vi "varun weather simu.vi"() -> ()   [LabVIEW 2021]
panel:
  in  "stop":bool
  out "Temp Status":string
  out "Freeze Warning":bool
  out "Heat Stroke Warning":bool
  out "Current Temp":dbl
  in  "Temp":dbl
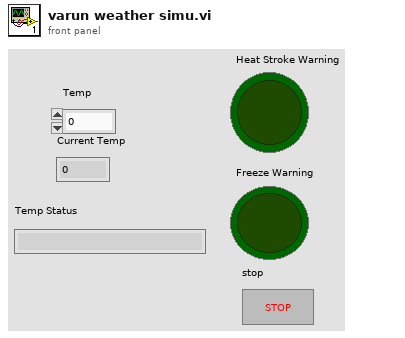
[diagram p1: front panel]
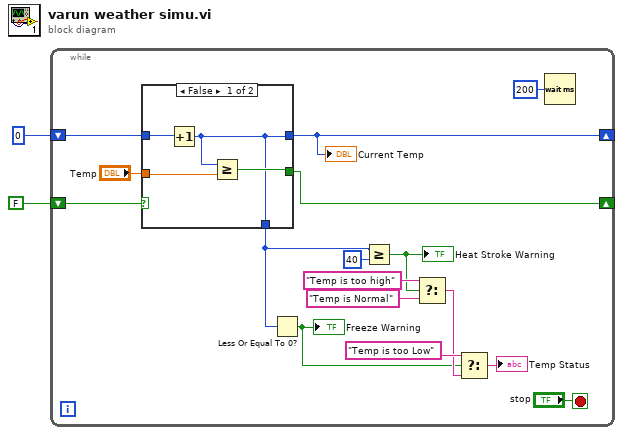
[diagram p0: block diagram]
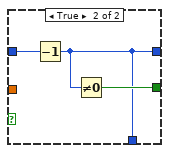
[diagram p2: hidden frame]
diagram:
  n1 = while {
    shift-right: [w15] -> _
    shift-left: 0 -> [w18]
    shift-right: [w16] -> _
    shift-left: FALSE -> [w17]
    stop <- "stop" stop-if-true
    n2 = case shown="False" w17 {
      tunnel: w18 -> [w22 w25]
      tunnel: [w21 w24] -> w16
      tunnel: [w19 w23] -> w15
      tunnel: "Temp" -> [w20 _]
      tunnel: [w19 w23] -> w7
      frame False {
        n3 = Increment(x=w22) -> (x+1=w19:i32)
        n4 = Greater Or Equal?(x=w19, y=w20) -> (x >= y?=w21:bool)
      }
      frame True {
        n5 = Decrement(x=w25) -> (x-1=w23:i32)
        n6 = Not Equal To 0?(x=w23) -> (x != 0?=w24:bool)
      }
    }
    "Current Temp" <- w15
    n7 = Less Or Equal To 0?(x=w7) -> (x <= 0?=w5:bool)
    "Freeze Warning" <- w5
    n8 = Greater Or Equal?(x=w7, y=40) -> (x >= y?=w6:bool)
    "Heat Stroke Warning" <- w6
    n9 = Select(t="Temp is too high", s=w6, f="Temp is Normal") -> (s? t:f=w12:string)
    n10 = Select(t="Temp is too Low", s=w5, f=w12) -> (s? t:f=→"Temp Status":string)
    n11 = Wait (ms)(milliseconds to wait=u32 200 ("millisecond timer value")) -> ()  [unwired: 1 out]
  }
